vi "Salidas.vi"(11 "Class 2.lvclass":refnum<class "Class 2.lvclass">) -> (3 "Class 2.lvclass 2":refnum<class "Class 2.lvclass">)   [LabVIEW 2019, in "Class 2.lvclass"]
uses:
  Class 2.lvclass
  Class 2.lvclass/Class 2.ctl
  Datos Out.vi
  Datos In.vi
panel:
  out "MAQ DE ESTADOS":T1
  out "SALIDAS.SMAC DISTANCIA":dbl
  out "SALIDAS.SMAC g":dbl
  out "SALIDAS.MENSAJES":string
  out "SALIDAS.SAMAC AVANZANDO":bool
  out "SALIDAS.SEMAC RETORNANDO":bool
  out "SALIDAS.CILINDRO 2":bool
  out "SALIDAS.CILINDRO 1":bool
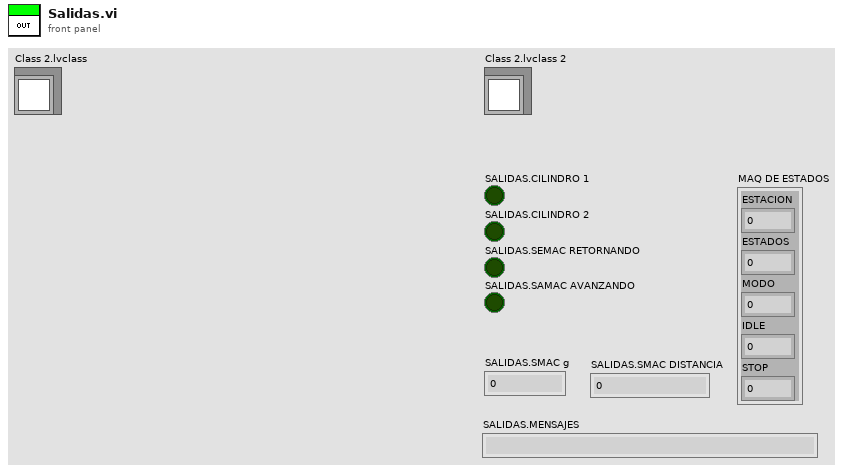
[diagram p1: front panel]
types:
  T1 = cluster{"ESTACION":i32, "ESTADOS":i16, "MODO":i16, "IDLE":i16, "STOP":i16}
  T2 = cluster{"SALIDAS.CILINDRO 1":bool, "SALIDAS.CILINDRO 2":bool, "SALIDAS.SEMAC RETORNANDO":bool, "SALIDAS.SAMAC AVANZANDO":bool, "Auto(off)/Manual(on)":bool, "HOME_CILINDRO_1":bool, "HOME_CILINDRO_2":bool, "AVANCE_CILINDRO_1":bool, "AVANCE_CILINDRO_2":bool, "PIEZA_EN_NIDO":bool, "BIMANUAL 2":bool, "BIMANUAL1":bool, "SIN CAMBIOS":bool, "CON  CAMBIOS":bool, "TESTER":bool, "MAQUINA EN ORIGEN":bool, "FALLA PRESENTE":bool}
  T3 = cluster{"Test":bool, "CILINDRO _1":bool, "CILINDRO _2":bool, "SMAC_RETORNANDO":bool, "SMAC_AVANZANDO":bool, "MANUAL":bool, "EST_1":bool, "EST_2":bool, "EST_3":bool, "MOVER A ORIGEN":bool, "RESET":bool, "PARO":bool, "INICIO":bool, "DATA_CONTROL":cluster{"ESTACION_1":cluster{"ACEPTADA":bool, "MAXIMO":dbl, "MINIMO":dbl, "LECTURA":dbl}, "ESTACION_2":cluster{"ACEPTADA":bool, "MAXIMO":dbl, "MINIMO":dbl, "LECTURA":dbl}, "ESTACION_3":cluster{"ACEPTADA":bool, "MAXIMO":dbl, "MINIMO":dbl, "LECTURA":dbl}}}
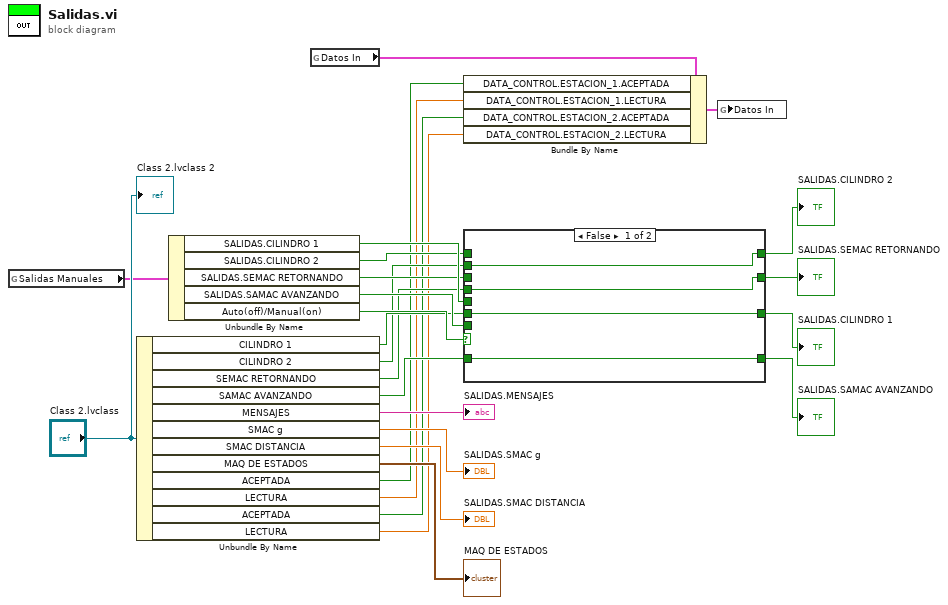
[diagram p0: block diagram]
diagram:
  n1 = global read "Datos Out.vi" "Salidas Manuales"() -> (w7:T2)
  n2 = Unbundle By Name("Class 2.lvclass") -> ("CILINDRO 1"=w16:bool, "CILINDRO 2"=w15:bool, "SEMAC RETORNANDO"=w14:bool, "SAMAC AVANZANDO"=w13:bool, "MENSAJES"=→"SALIDAS.MENSAJES":string, "SMAC g"=→"SALIDAS.SMAC g":dbl, "SMAC DISTANCIA"=→"SALIDAS.SMAC DISTANCIA":dbl, "MAQ DE ESTADOS"=→"MAQ DE ESTADOS":T1, "ACEPTADA"=w4:bool, "LECTURA"=w3:dbl, "ACEPTADA"=w2:bool, "LECTURA"=w1:dbl)
  n3 = Unbundle By Name(w7) -> ("SALIDAS.CILINDRO 1"=w20:bool, "SALIDAS.CILINDRO 2"=w19:bool, "SALIDAS.SEMAC RETORNANDO"=w18:bool, "SALIDAS.SAMAC AVANZANDO"=w17:bool, "Auto(off)/Manual(on)"=w21:bool)
  n4 = global read "Datos In.vi" "Datos In"() -> (w5:T3)
  n5 = Bundle By Name(cluster=w5, "DATA_CONTROL.ESTACION_1.ACEPTADA"=w4, "DATA_CONTROL.ESTACION_1.LECTURA"=w3, "DATA_CONTROL.ESTACION_2.ACEPTADA"=w2, "DATA_CONTROL.ESTACION_2.LECTURA"=w1) -> (w6:T3)
  n6 = case shown="False" w21 {
    tunnel: w20 -> [_ w33]
    tunnel: w19 -> [_ w32]
    tunnel: w18 -> [_ w31]
    tunnel: w17 -> [_ w30]
    tunnel: w16 -> [w29 _]
    tunnel: w15 -> [w28 _]
    tunnel: w14 -> [w27 _]
    tunnel: w13 -> [w26 _]
    tunnel: [w29 w33] -> w12
    tunnel: [w28 w32] -> w11
    tunnel: [w27 w31] -> w10
    tunnel: [w26 w30] -> w9
    frame False {
    }
    frame True {
    }
  }
  "SALIDAS.CILINDRO 1" <- w12
  "SALIDAS.CILINDRO 2" <- w11
  "SALIDAS.SEMAC RETORNANDO" <- w10
  "SALIDAS.SAMAC AVANZANDO" <- w9
  n7 = global write "Datos In.vi" "Datos In"(w6) -> ()
  "Class 2.lvclass 2" <- "Class 2.lvclass"
